vi "New Report Line.vi"(0 "report in":refnum<class "NI_HTML.lvclass">, 9 "number of lines (1)":i32=1, 11 "error in (no error)":errorcluster) -> (4 "report out":refnum<class "NI_HTML.lvclass">, 15 "error out":errorcluster)   [LabVIEW 2017, in "NI_HTML.lvclass"]
doc: "Starts a new line in the report."
uses:
  <vilib>/Utility/NIReport.llb/HTML/NI_HTML.lvclass
  <vilib>/Utility/NIReport.llb/HTML/NI_HTML.lvclass/NI_HTML.ctl
  <vilib>/Utility/NIReport.llb/NI_ReportGenerationCore.lvlib
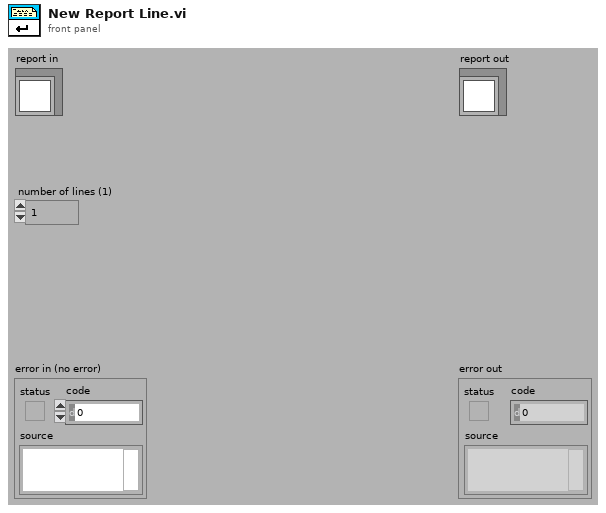
[diagram p1: front panel]
types:
  T1 = typedef "NI_ReportGenerationCore.lvlib/HTML Report Data.ctl" = cluster{"Body Text":string, "Font Tag":string, "Title Text":string, "Header Text":string, "Footer Text":string, "Image List":path[]}
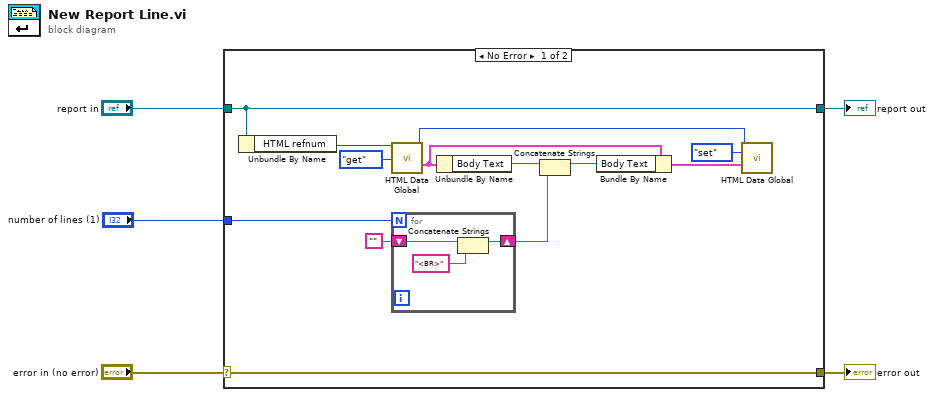
[diagram p0: block diagram]
diagram:
  n1 = case shown="No Error" "error in (no error)" {
    selector: "error in (no error)" -> [w18 w23]
    tunnel: [w18 w23] -> w4
    tunnel: [w11 w22] -> w2
    tunnel: "report in" -> [w11 w22]
    tunnel: "number of lines (1)" -> [w15 _]
    frame No Error {
      n2 = Unbundle By Name(w11) -> ("HTML refnum"=w14:u32)
      n3 = call <vilib>:"HTML Data Global.vi"("HTML refnum"=w14, "menu"=enum16{"init", "get", "set", "delete"}."get") -> ("HTML refnum out"=w7:u32, "HTML report data out"=w8:T1)  [unwired: 1 in, 11 out]
      n4 = for {
        N: w15 -> [_]
        shift-right: [w21] -> w16
        shift-left: "" ("Empty String Constant") -> [w20]
        n5 = Concatenate Strings(w20, "<BR>") -> (w21:string)
      }
      n6 = Unbundle By Name(w8) -> ("Body Text"=w12:string)
      n7 = Concatenate Strings(w12, w16) -> (w10:string)
      n8 = Bundle By Name(cluster=w8, "Body Text"=w10) -> (w9:T1)
      n9 = call <vilib>:"HTML Data Global.vi"("HTML refnum"=w7, "menu"=enum16{"init", "get", "set", "delete"}."set", "HTML report data in"=w9) -> ()  [unwired: 13 out]
    }
    frame Error {
    }
  }
  "error out" <- w4
  "report out" <- w2
